vi "Hold System Liste.vi"(1 "Action(GET)":enum16{"GET", "SET"}(ring), 7 "Loop Type in":variant, 11 "error in (no error)":errorcluster) -> (8 "Loops":string[](array[string]), 15 "error out":errorcluster)   [LabVIEW 2011]
uses:
  <vilib>/Utility/VariantDataType/GetNumericInfo.vi
  <vilib>/Utility/VariantDataType/VariantType.lvlib
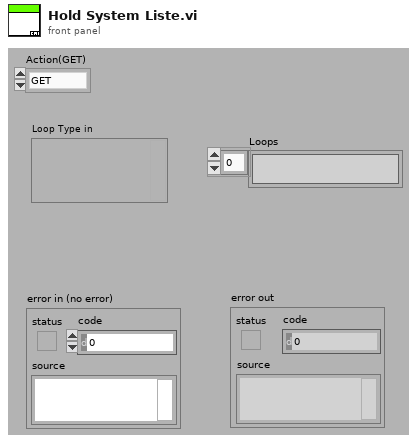
[diagram p1: front panel]
types:
  T1 = typedef "VariantType.lvlib/Type.ctl" = enum8{"Invalid Type", "Void", "I8", "I16", "I32", "I64", "U8", "U16", "U32", "U64", "Single Float", "Double Float", "Extended Float", "Single Complex", "Double Complex", "Extended Complex", "Enum U8", "Enum U16", "Enum U32", "Enum U64", "Single Float With Unit", "Double Float With Unit", "Extended Float With Unit", "Single Complex with Unit", "Double Complex with Unit", "Extended Complex with Unit", "Boolean", "String", "Path", "Picture", "Tag", "Array", "Cluster", "Variant", "LV Variant", "Waveform", "Timestamp", "Digital Waveform", "Digital Data", "ExpressData", "Refnum", "External Data", "VI", "Poly VI", "LabVIEW Class Instance", "Fixed Point"}
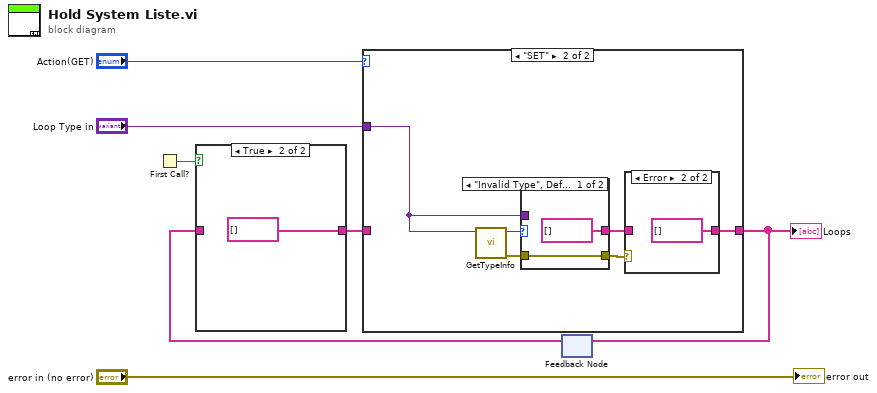
[diagram p0: block diagram]
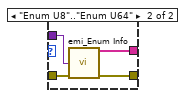
[diagram p5: hidden frame]
diagram:
  n1 = First Call?() -> (First Call?: T/F=w4:bool)
  n2 = feedback #1() -> (w5:string[])  [unwired: 1 in]
  n3 = case shown="True" w4 {
    tunnel: w5 -> [w8 _]
    tunnel: [w8 string[] [] ("Text Elements")] -> w2
    frame False {
    }
    frame True {
    }
  }
  n4 = case shown="\"SET\"" "Action(GET)" {
    tunnel: [w10 w12] -> w3
    tunnel: w2 -> [w10 _]
    tunnel: "Loop Type in" -> [_ w14]
    frame "GET", Default {
    }
    frame "SET" {
      n5 = call <vilib>:"GetTypeInfo.vi"("Variant"=w14) -> ("error out"=w15:errorcluster, "Type Enum"=w16:T1)  [unwired: 6 in, 3 out]
      n6 = case shown="\"Invalid Type\", Default" w16 {
        tunnel: w14 -> [_ w24]
        tunnel: w15 -> [w19 w23]
        tunnel: [string[] [] ("Text Elements") w22] -> w11
        tunnel: [w19 w21] -> w13
        frame "Invalid Type", Default {
        }
        frame "Enum U8".."Enum U64" {
          n7 = call "emi_Enum Info.vi"("Enum"=w24, "error in (no error)"=w23) -> ("Text Elements"=w22:string[], "error out"=w21:errorcluster)  [unwired: 10 in, 2 out]
        }
      }
      n8 = case shown="Error" w13 {
        tunnel: [w17 string[] [] ("Text Elements")] -> w12
        tunnel: w11 -> [w17 _]
        frame No Error {
        }
        frame Error {
        }
      }
    }
  }
  "Loops" <- w3
  n9 = feedback-in #1(w3) -> ()
  "error out" <- "error in (no error)"
